vi "FUG_PowerSupply.CreateServices.vi"(0 "i ref in":refnum<vi>, 5 "error in(no error)":errorcluster) -> (14 "i ref out":refnum<vi>, 19 "error out":errorcluster)   [LabVIEW 2014, in "FUG_PowerSupply.lvlib"]
doc: "This VI Creates two kinds of Services.\n\n1. Monitor services For the GUI, all Values there, are not-Raw Values.\n2. Set - Services for the DSCIntProc, all(most) values there are raw-values."
uses:
  FUG_PowerSupply.lvlib
  CSlibraries-extern/DimLVEvent/LVDimInterface/LVDimInterface.lvlib
  CS_Core/CSSystem/CSSystemLib/CSSystemLib.lvlib
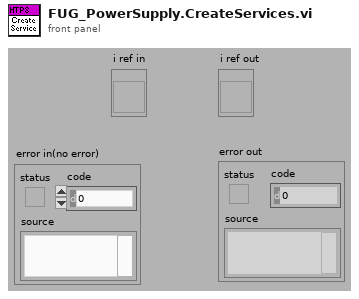
[diagram p1: front panel]
types:
  T1 = typedef "FUG_PowerSupply.lvlib/FUG_PowerSupply.i attribute.ctl" = cluster{"Type":string, "Elektrode Name":string, "CALC_FACTOR_SET_VOLTAGE":dbl, "CALC_FACTOR_GET_VOLTAGE":dbl, "CALC_FACTOR_GET_CURRENT":dbl, "CALC_FACTOR_SET_CURRENT ":dbl, "REG_VALUE":dbl, "Sign":bool, "setVoltID":i32, "setCurrentID":i32, "setPowerOnID":i32, "MaxVoltage":dbl}
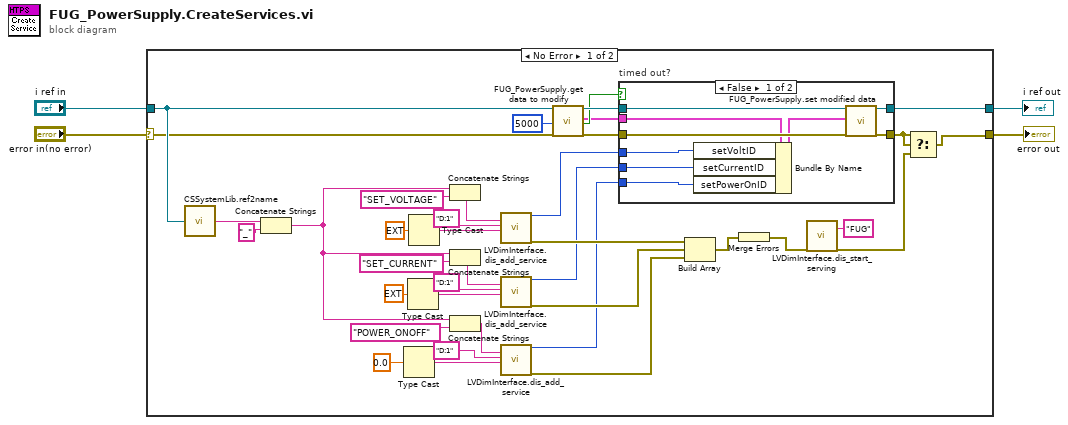
[diagram p0: block diagram]
diagram:
  n1 = case shown="No Error" "error in(no error)" {
    selector: "error in(no error)" -> [w11 w55]
    tunnel: [w15 w55] -> w1
    tunnel: "i ref in" -> [w12 w54]
    tunnel: [w42 w54] -> w2
    frame No Error {
      n2 = call "CSSystemLib.ref2name.vi"("obj refnum"=w12) -> ("name"=w22:string)
      n3 = Concatenate Strings(w22, "_" ("string")) -> (w23:string)
      n4 = Type Cast(x=0.0) -> (*(type *) &x=w28:string)  [unwired: 1 in]
      n5 = Type Cast(x=ext 0.0) -> (*(type *) &x=w33:string)  [unwired: 1 in]
      n6 = Type Cast(x=ext 0.0) -> (*(type *) &x=w38:string)  [unwired: 1 in]
      n7 = Concatenate Strings(w23, "SET_VOLTAGE") -> (w36:string)
      n8 = Concatenate Strings(w23, "SET_CURRENT" ("serviceName")) -> (w31:string)
      n9 = Concatenate Strings(w23, "POWER_ONOFF" ("serviceName")) -> (w26:string)
      n10 = call "LVDimInterface.dis_add_service.vi"("serviceName"=w36, "typeDescriptor"="D:1", "data"=w38) -> ("my_serviceID"=w7:i32, "error out"=w21:errorcluster)  [unwired: 15 in]
      n11 = call "LVDimInterface.dis_add_service.vi"("serviceName"=w31, "typeDescriptor"="D:1", "data"=w33) -> ("my_serviceID"=w6:i32, "error out"=w20:errorcluster)  [unwired: 15 in]
      n12 = call "LVDimInterface.dis_add_service.vi"("serviceName"=w26, "typeDescriptor"="D:1", "data"=w28) -> ("my_serviceID"=w5:i32, "error out"=w19:errorcluster)  [unwired: 15 in]
      n13 = call "FUG_PowerSupply.get data to modify.vi"("i ref in"=w12, "ms timeout (10000)"=5000, "error in (no error)"=w11) -> ("i ref out"=w18:refnum<vi>, "i attribute"=w10:T1, "timed out"=w13:bool, "error out"=w17:errorcluster)  [unwired: 13 in]
      n14 = case "timed out?" shown="False" w13 {
        tunnel: [w51 w53] -> w42
        tunnel: w18 -> [w50 w53]
        tunnel: w17 -> [w49 w52]
        tunnel: [w48 w52] -> w16
        tunnel: w10 -> [w47 _]
        tunnel: w7 -> [w45 _]
        tunnel: w6 -> [w44 _]
        tunnel: w5 -> [w43 _]
        frame False {
          n15 = Bundle By Name(cluster=w47, "setVoltID"=w45, "setCurrentID"=w44, "setPowerOnID"=w43) -> (w46:T1)
          n16 = call "FUG_PowerSupply.set modified data.vi"("i ref in"=w50, "i attribute"=w46, "error in (no error)"=w49) -> ("i ref out"=w51:refnum<vi>, "error out"=w48:errorcluster)  [unwired: 15 in]
        }
        frame True {
        }
      }
      n17 = Build Array(w21, w20, w19) -> (w25:errorcluster[])
      n18 = Merge Errors(w25) -> (w9:errorcluster)
      n19 = call "LVDimInterface.dis_start_serving.vi"("serverName"="FUG", "error in (no error)"=w9) -> ("error out"=w8:errorcluster)  [unwired: 16 in, 1 out]
      n20 = Select(t=w16, s=w16, f=w8) -> (s? t:f=w15:errorcluster)
    }
    frame Error {
    }
  }
  "error out" <- w1
  "i ref out" <- w2
